vi "Flush All FIFOs.vi"(8 "Error In":errorcluster, 11 "FPGA Ref":T1) -> (0 "Error Out":errorcluster)   [LabVIEW 2017]
doc: "Stops the acquisition."
uses:
  RIG-SPECIFIC FILES/FPGA Refs/FPGA Ref.ctl
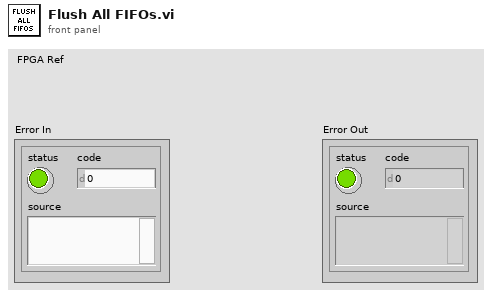
[diagram p1: front panel]
types:
  T1 = typedef "FPGA Ref.ctl" = refnum<k20>
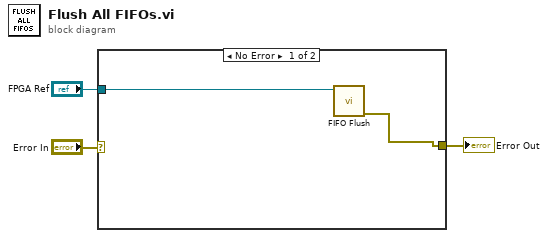
[diagram p0: block diagram]
diagram:
  n1 = case shown="No Error" "Error In" {
    selector: "Error In" -> [_ w6]
    tunnel: [w4 w6] -> w2
    tunnel: "FPGA Ref" -> [w5 _]
    frame No Error {
      n2 = call "FIFO Flush.vi"("FPGA VI Ref"=w5) -> ("Error Out"=w4:errorcluster)  [unwired: 8 in, 2 out]
    }
    frame Error {
    }
  }
  "Error Out" <- w2
